vi "Set Windows Debug Options.vi"(8 "error in":errorcluster, 9 "show threads":bool, 10 "show error dialog":bool, 11 "data sharing framework custom device in":T1 format="%.0x") -> (0 "error out":errorcluster, 3 "data sharing framework custom device out":T1 format="%.0x")   [LabVIEW 2017, in "Data Sharing Framework Custom Device Scripting.lvlib"]
doc: "Writes the <b>show error dialog</b> and <b>show threads</b> options. These options are available for Windows targets."
uses:
  Data Sharing Framework Custom Device Scripting.lvlib
  <vilib>/NI Veristand/Custom Device API/Custom Device Item Ref.ctl
  Shared/DSF Shared.lvlib
  System Explorer/DSF System Explorer.lvlib
  <vilib>/NI VeriStand/Custom Device API/Custom Device API.lvlib
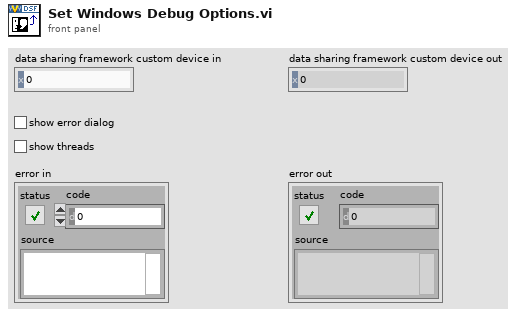
[diagram p1: front panel]
types:
  T1 = typedef "Custom Device API.lvlib/Custom Device Item Ref.ctl" = u64
  T2 = typedef "DSF Core.lvlibp/Framework.lvclass/Framework Options.ctl" = cluster{"FIFO Options":T3, "Thread Options":T4, "Plugin Options":T5, "Performance Options":T6, "Data Server Options":T7}
  T3 = typedef "DSF Core.lvlibp/Framework.lvclass/DSF FIFO Options.ctl" = cluster{"Infinite Timeouts":bool}
  T4 = typedef "DSF Core.lvlibp/Thread.lvclass/Thread Options.ctl" = cluster{"Show FP On Call":bool, "Close FP After Call":bool, "Allow Debugging":bool}
  T5 = typedef "DSF Core.lvlibp/Framework.lvclass/DSF Plugin Options.ctl" = cluster{"Default Components":bool}
  T6 = typedef "DSF Core.lvlibp/DSF Performance Options.ctl" = cluster{"Measure Period":bool, "Measure Rx/Tx Duration":bool}
  T7 = typedef "DSF Core.lvlibp/Framework.lvclass/Data Server Options.ctl" = cluster{"Enable Data Server":bool, "Period":u32}
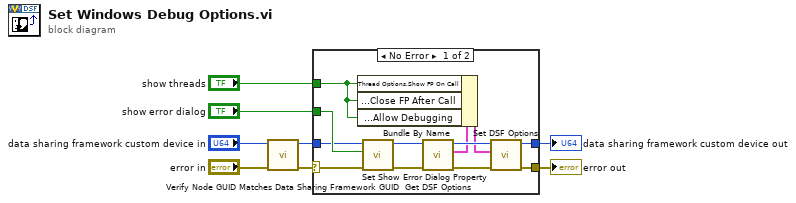
[diagram p0: block diagram]
diagram:
  n1 = call "Verify Node GUID Matches Data Sharing Framework GUID.vi"("error in"="error in", "data sharing framework custom device in"="data sharing framework custom device in") -> ("error out"=w3:errorcluster, "data sharing framework custom device out"=w4:T1)  [unwired: 8 in]
  n2 = case shown="No Error" w3 {
    selector: w3 -> [w9 w21]
    tunnel: [w18 w22] -> w8
    tunnel: [w17 w21] -> w7
    tunnel: "show threads" -> [w16 _]
    tunnel: "show error dialog" -> [w13 _]
    tunnel: w4 -> [w10 w22]
    frame No Error {
      n3 = call "Set Show Error Dialog Property.vi"("error in (no error)"=w9, "show error dialog"=w13, "Item Ref in"=w10) -> ("error out"=w11:errorcluster, "Item Ref out"=w12:T1)  [unwired: 7 in]
      n4 = call "Get DSF Options.vi"("error in (no error)"=w11, "Item Ref in"=w12) -> ("error out"=w19:errorcluster, "options"=w15:T2, "Item Ref out"=w20:T1)  [unwired: 7 in]
      n5 = Bundle By Name(cluster=w15, "Thread Options.Show FP On Call"=w16, "Thread Options.Close FP After Call"=w16, "Thread Options.Allow Debugging"=w16) -> (w14:T2)
      n6 = call "Set DSF Options.vi"("error in (no error)"=w19, "options"=w14, "Item Ref in"=w20) -> ("error out"=w17:errorcluster, "Item Ref out"=w18:T1)  [unwired: 7 in]
    }
    frame Error {
    }
  }
  "data sharing framework custom device out" <- w8
  "error out" <- w7
